vi "get_cpu_string.vi"() -> ()   [LabVIEW 2026]
uses:
  hello_cpu_lib/target/release/hello_cpu_lib.dll
panel:
  out "cpu_string_handle":string
  out "cpu_string_pointer":string
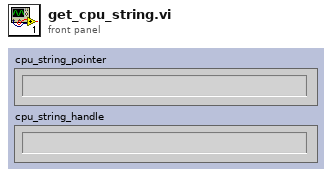
[diagram p1: front panel]
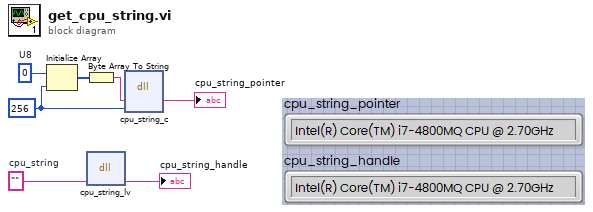
[diagram p0: block diagram]
diagram:
  w1 = 256 ("dimension size")
  w6 = u8 0  # U8
  w7 = ""  # cpu_string
  n1 = Initialize Array(w6, w1) -> (w5:u8[])
  n2 = Byte Array To String(unsigned byte array=w5) -> (string=w4:string)
  n3 = dll-call lib="C:/Users/Andrey/Desktop/hello_cpu_lib/target/release/hello_cpu_lib.dll" fn="cpu_string_lv"("cpu_string_handle"=w7) -> ("cpu_string_handle"=→"cpu_string_handle":string)  [unwired: 4 in, 2 out]
  n4 = dll-call lib="C:/Users/Andrey/Desktop/hello_cpu_lib/target/release/hello_cpu_lib.dll" fn="cpu_string_c"("cpu_string_pointer"=w4, "length"=w1) -> ("cpu_string_pointer"=→"cpu_string_pointer":string)  [unwired: 5 in, 2 out]
